vi "Read Collision Grid Info.vi"(8 "error in (no error)":errorcluster, 11 "Collider in":refnum<class "Collider.lvclass">) -> (0 "error out":errorcluster, 2 "Collision Grid Info":T1, 3 "Collider out":refnum<class "Collider.lvclass">)   [LabVIEW 2022 SP3, in "Collider.lvclass"]
uses:
  Collider.lvclass
  Collider.lvclass/Collider.ctl
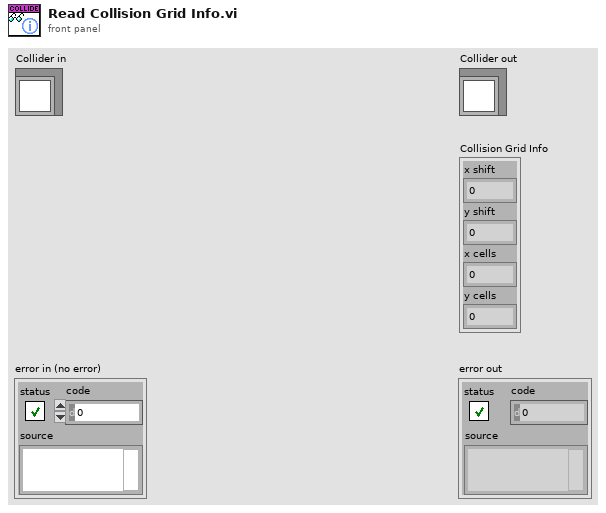
[diagram p1: front panel]
types:
  T1 = cluster{"x shift":i16, "y shift":i16, "x cells":i16, "y cells":i16}
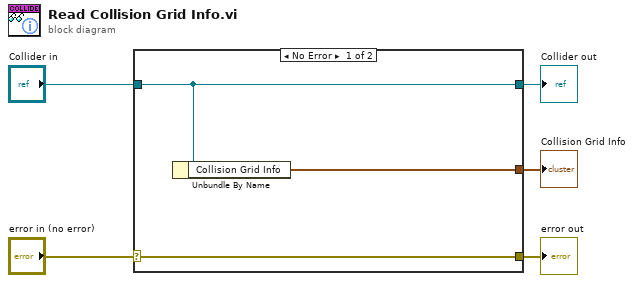
[diagram p0: block diagram]
diagram:
  n1 = case shown="No Error" "error in (no error)" {
    selector: "error in (no error)" -> [w8 w9]
    tunnel: [w8 w9] -> w4
    tunnel: [w7 w10] -> w2
    tunnel: "Collider in" -> [w7 w10]
    tunnel: [w6 _] -> w1
    frame No Error {
      n2 = Unbundle By Name(w7) -> ("Collision Grid Info"=w6:T1)
    }
    frame Error {
    }
  }
  "error out" <- w4
  "Collider out" <- w2
  "Collision Grid Info" <- w1
